vi "indentation constant.vi"() -> (0 "indentation":string)   [LabVIEW 2024, in "atsj peakcan basic.lvlib"]
uses:
  atsj peakcan basic.lvlib
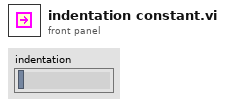
[diagram p1: front panel]
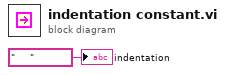
[diagram p0: block diagram]
diagram:
  "indentation" <- "     "
